vi "Initialize.vi"(8 "error in (no error)":errorcluster, 11 "MB in":refnum<class "Master CR.lvclass">) -> (0 "error out":errorcluster, 3 "MB out":refnum<class "Master CR.lvclass">)   [LabVIEW 2021, in "Master CR.lvclass"]
uses:
  Master CR.lvclass
  Master CR.lvclass/Master CR.ctl
  Modbus_v121c/Data Model/Device Data Model.lvclass
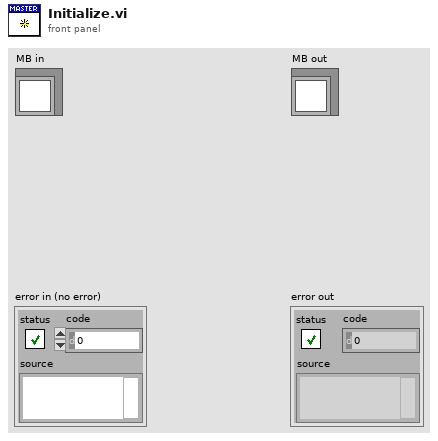
[diagram p1: front panel]
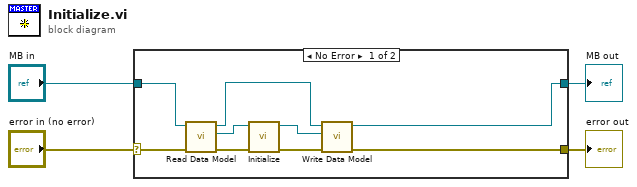
[diagram p0: block diagram]
diagram:
  n1 = case shown="No Error" "error in (no error)" {
    selector: "error in (no error)" -> [w7 w14]
    tunnel: [w5 w14] -> w3
    tunnel: [w6 w15] -> w1
    tunnel: "MB in" -> [w8 w15]
    frame No Error {
      n2 = call "Read Data Model.vi"("error in (no error)"=w7, "Master CR in"=w8) -> ("error out"=w12:errorcluster, "Data Model"=w13:refnum<class "Device Data Model.lvclass">, "Master CR out"=w9:refnum<class "Master CR.lvclass">)  [unwired: 7 in]
      n3 = call-dynamic "Initialize.vi"("error in"=w12, "device data model in"=w13) -> ("error out"=w11:errorcluster, "device data model out"=w10:refnum<class "Device Data Model.lvclass">)  [unwired: 8 in]
      n4 = call "Write Data Model.vi"("error in (no error)"=w11, "Data Model"=w10, "Master CR in"=w9) -> ("error out"=w5:errorcluster, "Master CR out"=w6:refnum<class "Master CR.lvclass">)  [unwired: 7 in]
    }
    frame Error {
    }
  }
  "error out" <- w3
  "MB out" <- w1
